vi "Write Scalar Boolean.vi"(8 "error in (no error)":errorcluster, 10 "value":bool, 11 "pointer in":u64) -> (0 "error out":errorcluster, 3 "pointer out":u64)   [LabVIEW 2013, in "Linux RT IPC.lvlib" / "Shared Memory.lvlib"]
uses:
  Shared Memory.lvlib
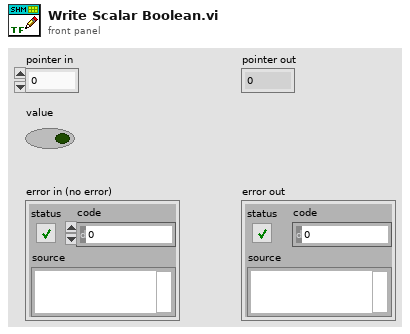
[diagram p1: front panel]
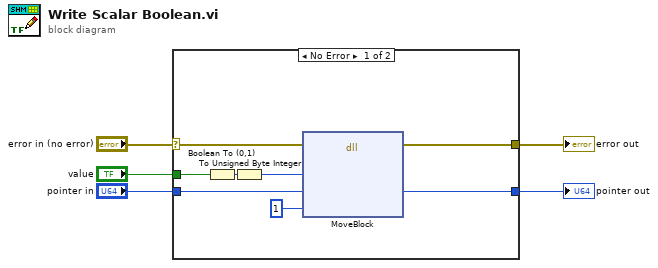
[diagram p0: block diagram]
diagram:
  n1 = case shown="No Error" "error in (no error)" {
    selector: "error in (no error)" -> [w10 w15]
    tunnel: [w9 w15] -> w5
    tunnel: "pointer in" -> [w8 w14]
    tunnel: "value" -> [w13 _]
    tunnel: [w7 w14] -> w2
    frame No Error {
      n2 = Boolean To (0,1)(Boolean=w13) -> (0, 1=w12:i16)
      n3 = To Unsigned Byte Integer(number=w12) -> (unsigned 8bit integer=w6:u8)
      n4 = dll-call lib="LabVIEW" fn="MoveBlock"(error in=w10, "data"=w6, "pointer"=w8, "size"=u64 1) -> (error out=w9:errorcluster, "pointer"=w7:u64)  [unwired: 5 in, 1 out]
    }
    frame Error {
    }
  }
  "error out" <- w5
  "pointer out" <- w2
